vi "BodeMagnitudePlot.vi"() -> ()   [LabVIEW 2014]
doc: "This program takes an input ai0 and outputs to ao0 and computes the gain for each frequency output and makes a bode plot of gain vs frequency\n\nBryan Ghahremani -SID: 1135515\nKenneth Heide -SID: 1269429"
uses:
  <vilib>/Analysis/NI_AALPro.lvlib
panel:
  out "output cluster":cluster{dbl, dbl}={2010.0, -15.491634603155624}
  out "XY Graph":cluster{"X":dbl, "Y":dbl}[](graph)=[{"X"=10.0, "Y"=-0.0047080348899403565}, {"X"=35.0, "Y"=-0.003709257179983122}, {"X"=60.0, "Y"=-0.05029100406630311}, {"X"=85.0, "Y"=-0.14241947780273567}, {"X"=110.0, "Y"=-0.27732723820353233}, {"X"=135.0, "Y"=-0.4513498324815396}, {"X"=160.0, "Y"=-0.6598382830123155}, {"X"=185.0, "Y"=-0.8972259660376873}, {"X"=210.0, "Y"=-1.159061177296015}, {"X"=235.0, "Y"=-1.440246337130124}, {"X"=260.0, "Y"=-1.7358609127537197}, {"X"=285.0, "Y"=-2.0425332852396867}, {"X"=310.0, "Y"=-2.3566088807116485}, {"X"=335.0, "Y"=-2.674880893698981}, {"X"=360.0, "Y"=-2.9949397528110406}, {"X"=385.0, "Y"=-3.3155129961066043}, {"X"=410.0, "Y"=-3.6341603558690276}, {"X"=435.0, "Y"=-3.9502266460161835}, {"X"=460.0, "Y"=-4.262712018743022}, {"X"=485.0, "Y"=-4.570092935282984}, {"X"=510.0, "Y"=-4.87284406838313}, {"X"=535.0, "Y"=-5.170724211598451}, {"X"=560.0, "Y"=-5.463099116811284}, {"X"=585.0, "Y"=-5.748783107240499}, {"X"=610.0, "Y"=-6.028528946596007}, {"X"=635.0, "Y"=-6.302647189167784}, {"X"=660.0, "Y"=-6.5721432790050285}, {"X"=685.0, "Y"=-6.834171913904894}, {"X"=710.0, "Y"=-7.090371713281786}, {"X"=735.0, "Y"=-7.3416273011431485}, {"X"=760.0, "Y"=-7.5868989154734585}, {"X"=785.0, "Y"=-7.827163309751207}, {"X"=810.0, "Y"=-8.061324224394575}, {"X"=835.0, "Y"=-8.291106357809463}, {"X"=860.0, "Y"=-8.517224689598507}, {"X"=885.0, "Y"=-8.736383636735445}, {"X"=910.0, "Y"=-8.952281601966432}, {"X"=935.0, "Y"=-9.163619976025302}, {"X"=960.0, "Y"=-9.370828828973718}, {"X"=985.0, "Y"=-9.572545787304016}, {"X"=1010.0, "Y"=-9.77174680689769}, {"X"=1035.0, "Y"=-9.966561607452972}, {"X"=1060.0, "Y"=-10.157934281705872}, {"X"=1085.0, "Y"=-10.344512651942333}, {"X"=1110.0, "Y"=-10.52778847968613}, {"X"=1135.0, "Y"=-10.708798945359103}, {"X"=1160.0, "Y"=-10.885045694318219}, {"X"=1185.0, "Y"=-11.059142893480757}, {"X"=1210.0, "Y"=-11.228936118016225}, {"X"=1235.0, "Y"=-11.39548494777671}, {"X"=1260.0, "Y"=-11.561144485008024}, {"X"=1285.0, "Y"=-11.722854283210967}, {"X"=1310.0, "Y"=-11.881508729379613}, {"X"=1335.0, "Y"=-12.0386358477381}, {"X"=1360.0, "Y"=-12.19224224607725}, {"X"=1385.0, "Y"=-12.342727119881442}, {"X"=1410.0, "Y"=-12.49260379809889}, {"X"=1435.0, "Y"=-12.639464444619646}, {"X"=1460.0, "Y"=-12.78342290745017}, {"X"=1485.0, "Y"=-12.925743605846321}, {"X"=1510.0, "Y"=-13.0645013776262}, {"X"=1535.0, "Y"=-13.201975367134448}, {"X"=1560.0, "Y"=-13.337674068487921}, {"X"=1585.0, "Y"=-13.472473094424931}, {"X"=1610.0, "Y"=-13.605575880571477}, {"X"=1635.0, "Y"=-13.732668265164325}, {"X"=1660.0, "Y"=-13.86182442913903}, {"X"=1685.0, "Y"=-13.988586966860417}, {"X"=1710.0, "Y"=-14.114891092781402}, {"X"=1735.0, "Y"=-14.23865591789995}, {"X"=1760.0, "Y"=-14.357096895061531}, {"X"=1785.0, "Y"=-14.479407734424017}, {"X"=1810.0, "Y"=-14.596759229922657}, {"X"=1835.0, "Y"=-14.712842064384104}, {"X"=1860.0, "Y"=-14.830106101526596}, {"X"=1885.0, "Y"=-14.943456212412961}, {"X"=1910.0, "Y"=-15.056645680005069}, {"X"=1935.0, "Y"=-15.164969739236767}, {"X"=1960.0, "Y"=-15.276803009879984}, {"X"=1985.0, "Y"=-15.386287510482878}, {"X"=2010.0, "Y"=-15.491634603155624}]
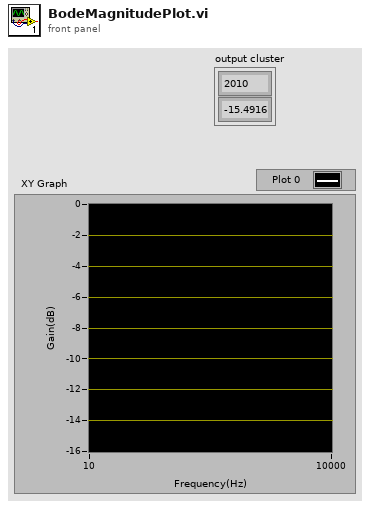
[diagram p1: front panel]
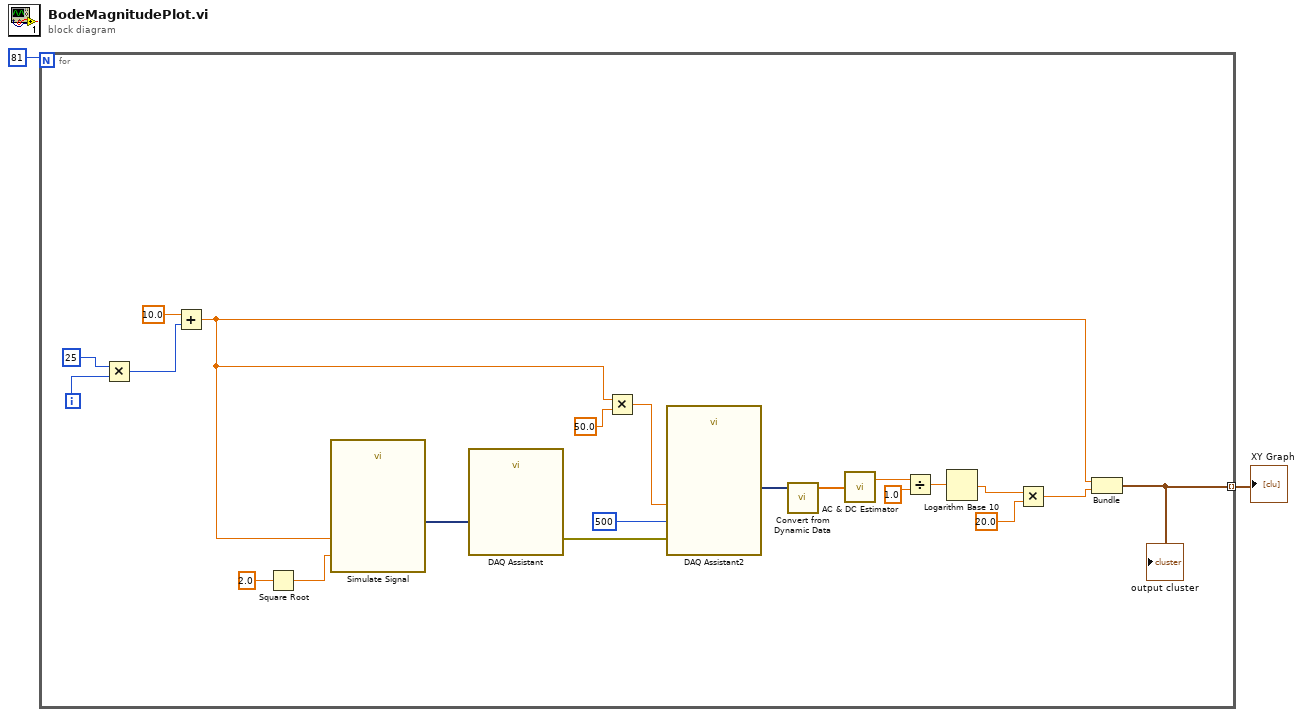
[diagram p0: block diagram]
diagram:
  n1 = for {
    N: 81 -> [_]
    tunnel: [w5] -> w1 mode=indexing
    i -> [w21]
    n2 = Multiply(x=25, y=w21) -> (x*y=w22:i32)
    n3 = Add(x=10.0, y=w22) -> (x+y=w7:dbl)
    n4 = Square Root(x=2.0) -> (sqrt(x)=w19:dbl)
    n5 = call "Simulate Signal"("Frequency"=w7, "Amplitude"=w19) -> ("Sine"=w16:dynamicdata)  [unwired: 12 in, 1 out]
    n6 = call "DAQ Assistant"("data"=w16) -> ("error out"=w14:errorcluster)  [unwired: 16 in, 2 out]
    n7 = Multiply(x=w7, y=50.0) -> (x*y=w13:dbl)
    n8 = call "DAQ Assistant2"("rate"=w13, "number of samples"=500, "error in"=w14) -> ("data"=w12:dynamicdata)  [unwired: 14 in, 2 out]
    n9 = call "Convert from Dynamic Data"("Dynamic Data Type"=w12) -> ("Array"=w11:dbl[])  [unwired: 3 in]
    n10 = call <vilib>:"AC & DC Estimator.vi"("Signal (V)"=w11) -> ("AC estimate (Vrms)"=w10:dbl)  [unwired: 1 out]
    n11 = Divide(x=w10, y=1.0) -> (x/y=w4:dbl)
    n12 = Logarithm Base 10(1:w4) -> (0:w3:dbl)
    n13 = Multiply(x=w3, y=20.0) -> (x*y=w6:dbl)
    n14 = Bundle(w7, w6) -> (w5:cluster{dbl, dbl})  [unwired: 1 in]
    "output cluster" <- w5
  }
  "XY Graph" <- w1
